vi "Add Task.vi"(8 "error in (no error)":errorcluster, 10 "Analog Configuration Parameters":T1, 11 "Analog Input in":refnum<class "Analog Input.lvclass">) -> (0 "error out":errorcluster, 3 "Analog Input out":refnum<class "Analog Input.lvclass">)   [LabVIEW 2021, in "Analog Input.lvlib" / "Analog Input.lvclass"]
uses:
  Analog Input.lvclass
  <vilib>/DAQmx/create/channels.llb/DAQmx Create Channel (AI-Voltage-Basic).vi
  Utilities/Analog Configuration Parameters.ctl
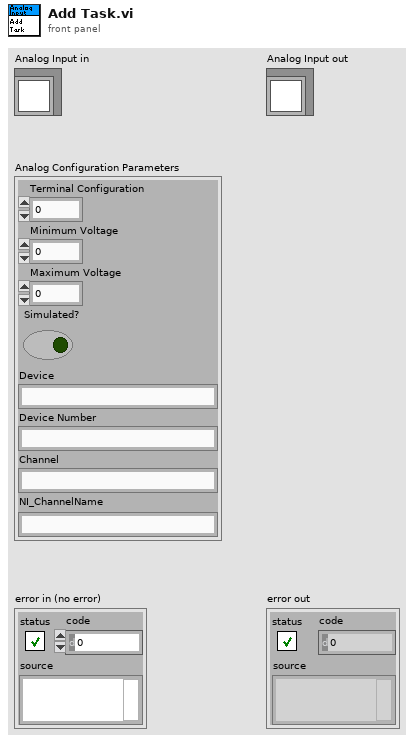
[diagram p1: front panel]
types:
  T1 = typedef "Analog Configuration Parameters.ctl" = cluster{"Terminal Configuration":i32, "Minimum Voltage":dbl, "Maximum Voltage":dbl, "Simulated?":bool, "Device":string, "Device Number":string, "Channel":string, "NI_ChannelName":string}
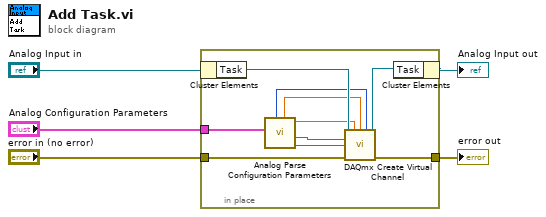
[diagram p0: block diagram]
diagram:
  n1 = in-place {
    in-place-border: "Analog Configuration Parameters" -> [w8]
    in-place-border: "error in (no error)" -> [w7]
    in-place-border: [w6] -> w1
    n2 = in-place-cluster #1("Analog Input in") -> ("Task"=w15:refnum<k21>)
    n3 = call "Analog Parse Configuration Parameters.vi"("Analog Configuration Parameters"=w8) -> ("name to assign"=w13:string, "physical channels"=w12:string, "Maximum Voltage"=w11:dbl, "Minimum Voltage"=w10:dbl, "Terminal Configuration"=w9:i32)  [unwired: 6 in]
    n4 = call-poly <vilib>:"DAQmx Create Virtual Channel.vi"("task in"=w15, "maximum value"=w11, "minimum value"=w10, "input terminal configuration"=w9, "physical channels"=w12, "name to assign"=w13, "error in"=w7) -> ("task out"=w14:refnum<k21>, "error out"=w6:errorcluster)  [unwired: 7 in]
    n5 = in-place-cluster #1("Task"=w14) -> (→"Analog Input out":refnum<class "Analog Input.lvclass">)
  }
  "error out" <- w1
